vi "Execute.vi"(8 "error in":errorcluster, 11 "Change O2 Valve in":refnum<class "Change O2 Valve.lvclass">) -> (0 "error out":errorcluster, 1 "Next Step?":bool, 2 "MSG":string, 3 "Change O2 Valve out":refnum<class "Change O2 Valve.lvclass">)   [LabVIEW 2015, in "Change O2 Valve.lvclass"]
uses:
  Change O2 Valve.lvclass
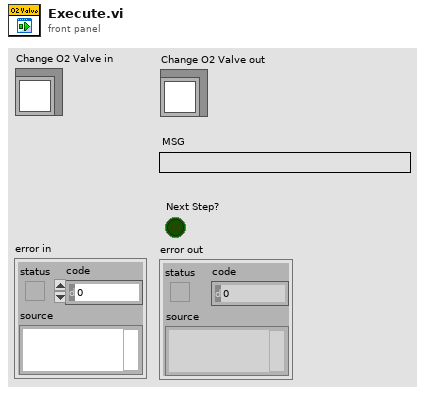
[diagram p1: front panel]
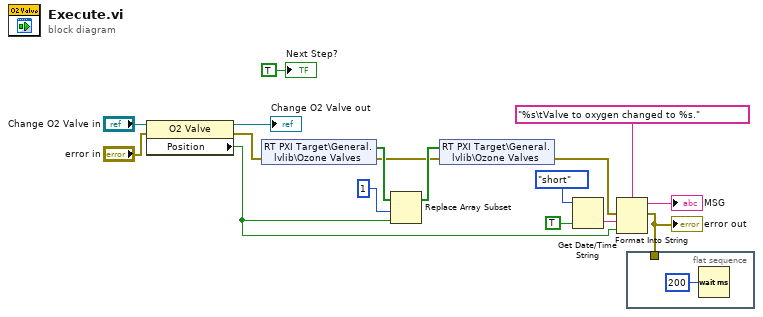
[diagram p0: block diagram]
diagram:
  n1 = property class="O2 Valve"(reference="Change O2 Valve in", error in="error in") -> (reference out=→"Change O2 Valve out":refnum<class "Change O2 Valve.lvclass">, error out=w3:errorcluster, "Position"=w7:bool)
  n2 = shared-variable "RT PXI Target\\General.lvlib\\Ozone Valves"(error in=w3) -> (w4:bool[], error out=w2:errorcluster)
  n3 = Replace Array Subset(array=w4, new element=w7, index=1) -> (w5:bool[])
  n4 = shared-variable "RT PXI Target\\General.lvlib\\Ozone Valves"(w5, error in=w2) -> (error out=w8:errorcluster)
  n5 = Get Date/Time String(date format (0)=enum16{"short", "long", "abbreviated"}."short", want seconds? (F)=TRUE) -> (time string=w12:string)  [unwired: 1 in, 1 out]
  n6 = Format Into String(format string="%s\tValve to oxygen changed to %s.", error in=w8, w12, w7) -> (resulting string=→"MSG":string, error out=w1:errorcluster)  [unwired: 1 in]
  "error out" <- w1
  n7 = flat-sequence {
    tunnel: w1 -> [_]
    frame #0 {
      n8 = Wait (ms)(milliseconds to wait=u32 200) -> ()  [unwired: 1 out]
    }
  }
  "Next Step?" <- TRUE ("Next Step?")
